vi "生产调试用上位机.vi"() -> ()   [LabVIEW 2016]
uses:
  <vilib>/Utility/miscctls.llb/LVPointTypeDef.ctl
  <vilib>/Utility/config.llb/NI_LVConfig.lvlib
panel:
  in  "隐藏":bool
  out "软件版本":string
  in  "报警查询":bool
  in  "日志查询":bool
  in  "主页按钮":bool
  in  "数据查询":bool
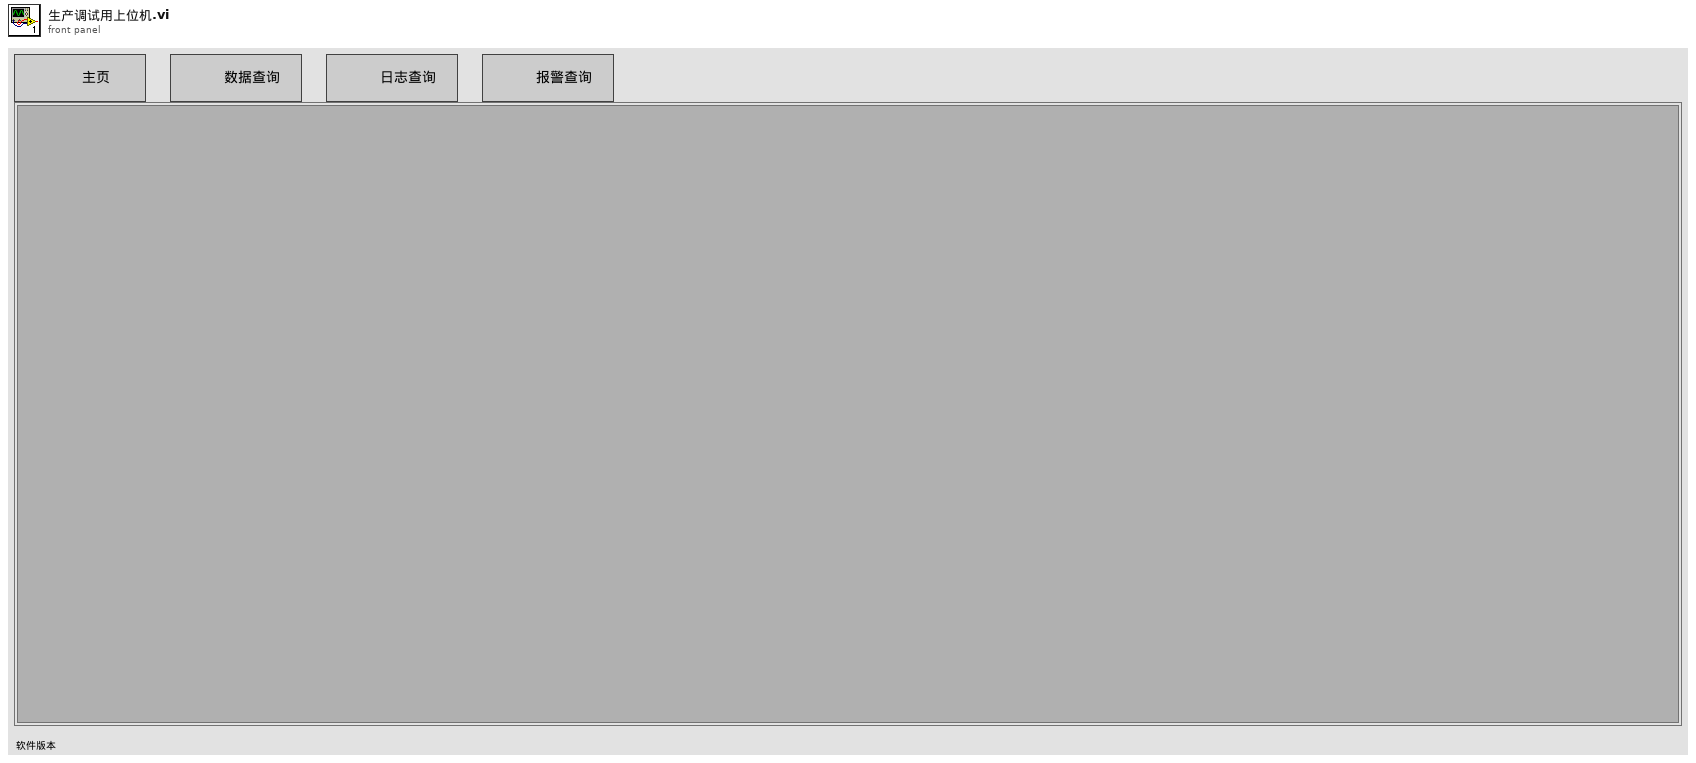
[diagram p1: front panel]
types:
  T1 = typedef "LVPointTypeDef.ctl" = cluster{"Horizontal":i16, "Vertical":i16}
  T2 = typedef "NI_LVConfig.lvlib/Config Data RefNum.ctl" = refnum<k1>
  T3 = enum32{"Bad", "Idle", "Run top level", "Running"}
  T4 = typedef "imagedata.ctl" = cluster{"image type":i32, "image depth":i32, "image":u8[], "mask":u8[], "colors":u32[], "Rectangle":cluster{"left":i16, "top":i16, "right":i16, "bottom":i16}}
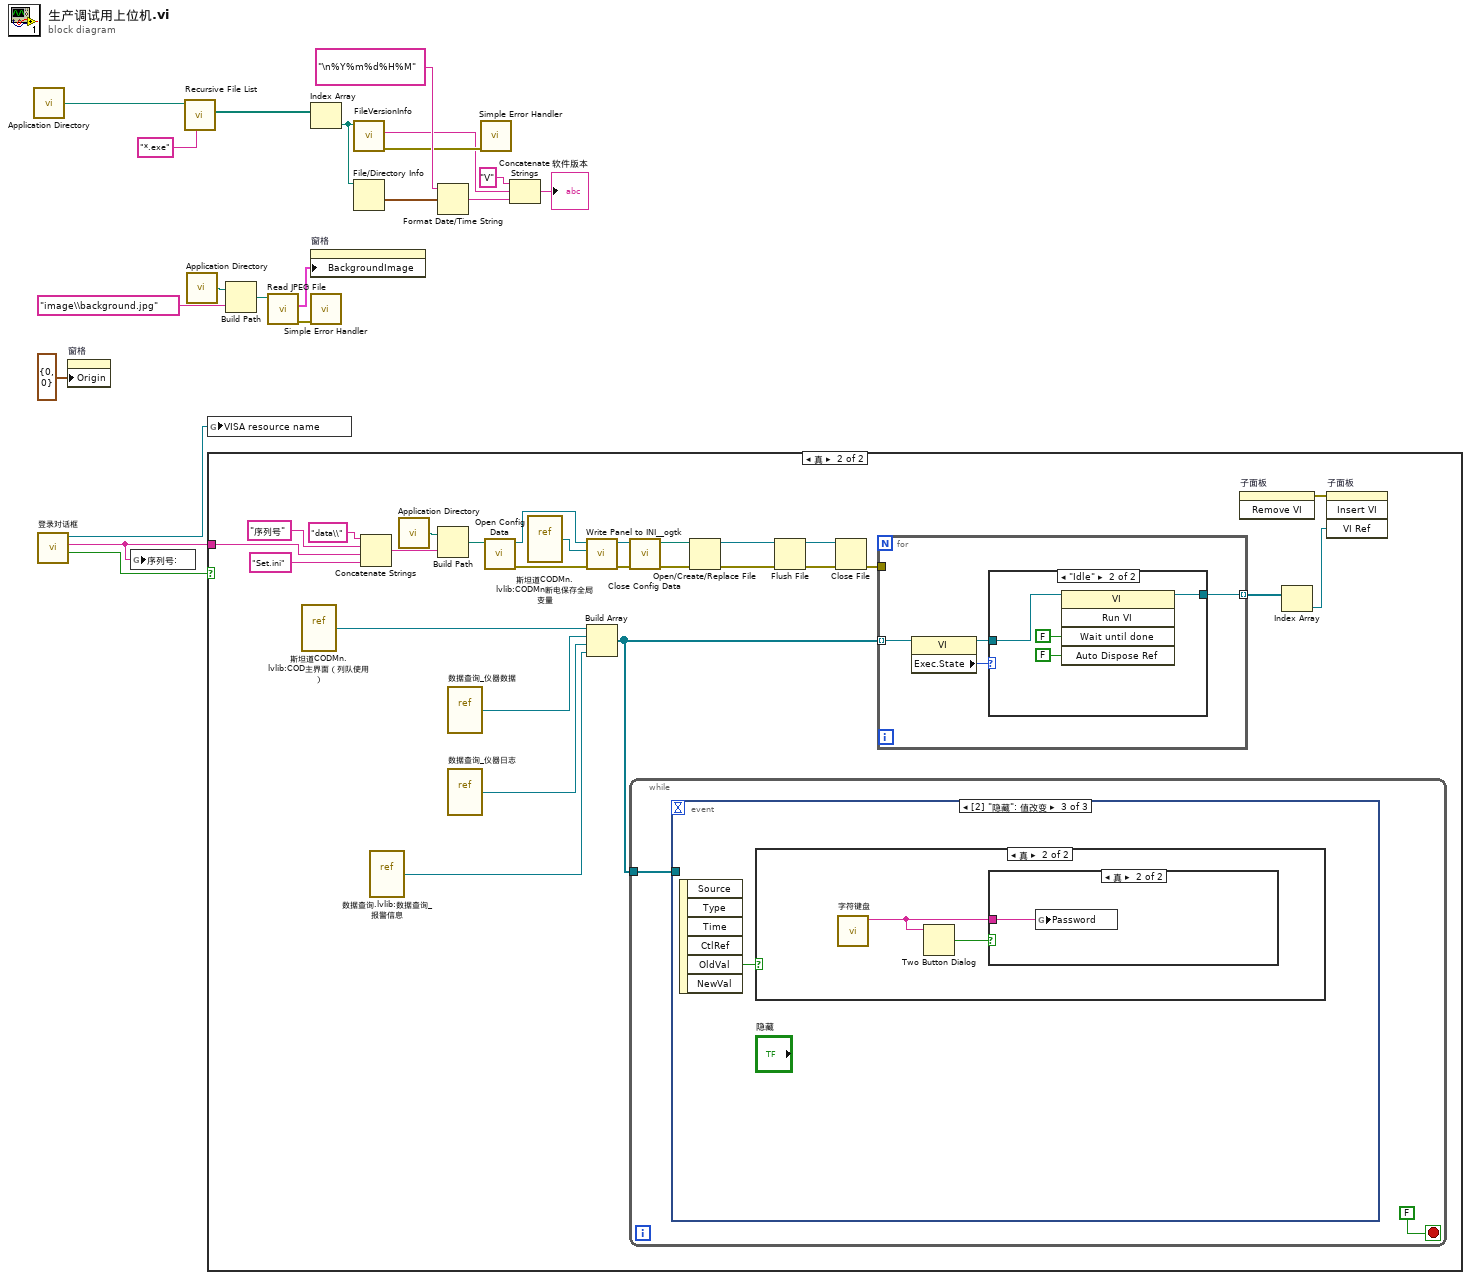
[diagram p0: block diagram]
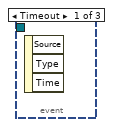
[diagram p4: hidden frame]
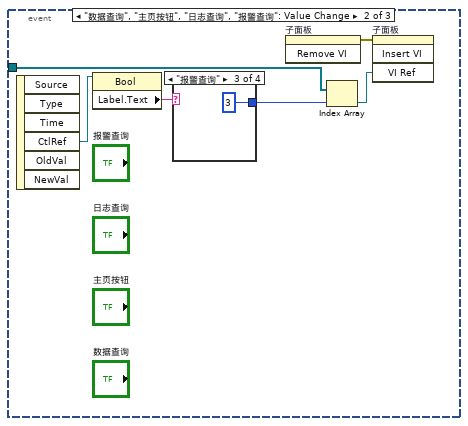
[diagram p5: hidden frame]
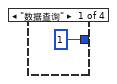
[diagram p6: hidden frame]
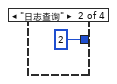
[diagram p7: hidden frame]
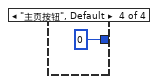
[diagram p8: hidden frame]
diagram:
  n1 = call <vilib>:"Application Directory.vi"() -> ("Application Directory"=w10:path)
  n2 = call "登录对话框.vi"() -> ("输出"=w15:bool, "序列号"=w12:string, "串口号"=w14:refnum<visa-resource-name>)  [unwired: 7 in]
  n3 = property on="窗格" class="Pane"("Origin"=T1 {"Horizontal"=0, "Vertical"=0} ("原点")) -> ()  [unwired: 2 in, 2 out]
  n4 = global write "COD内部交互全局.vi" "序列号:"(w12) -> ()
  n5 = call <vilib>:"Recursive File List.vi"("pattern"="*.exe", "Folder Path"=w10) -> ("All Files in Dir"=w2:path[])  [unwired: 5 in, 4 out]
  n6 = call <vilib>:"Application Directory.vi"() -> ("Application Directory"=w20:path)
  n7 = global write "CODMn断电保存全局变量.vi" "VISA resource name"(w14) -> ()
  n8 = case shown="真" w15 {
    tunnel: w12 -> [_ w38]
    frame False {
    }
    frame True {
      n9 = vi-ref "斯坦道CODMn.lvlib:COD主界面（列队使用）.vi"() -> (w47:refnum<vi>)
      n10 = Concatenate Strings("data\\" ("字符串"), "序列号" ("字符串"), w38, "Set.ini" ("名称或相对路径")) -> (w24:string)
      n11 = vi-ref "数据查询.lvlib:数据查询_报警信息.vi"() -> (w22:refnum<vi>)
      n12 = call <vilib>:"Application Directory.vi"() -> ("Application Directory"=w25:path)
      n13 = Build Path(base path=w25, name or relative path=w24) -> (appended path=w26:path)
      n14 = vi-ref "数据查询_仪器数据.vi"() -> (w46:refnum<vi>)
      n15 = vi-ref "数据查询_仪器日志.vi"() -> (w21:refnum<vi>)
      n16 = call <vilib>:"Open Config Data.vi"("configuration file path"=w26) -> ("error out"=w30:errorcluster, "refnum"=w27:T2)  [unwired: 8 in, 1 out]
      n17 = vi-ref "斯坦道CODMn.lvlib:CODMn断电保存全局变量.vi"() -> (w28:refnum<vi>)
      n18 = call <userlib>:"Write Panel to INI__ogtk.vi"("error in (no error)"=w30, "VI ref"=w28, "refnum"=w27) -> ("error out"=w31:errorcluster, "refnum out"=w29:T2)  [unwired: 7 in]
      n19 = Build Array(w47, w46, w21, w22) -> (w42:refnum<vi>[])
      n20 = call <vilib>:"Close Config Data.vi"("error in (no error)"=w31, "refnum"=w29) -> ("error out"=w36:errorcluster, "file path"=w37:path)  [unwired: 8 in]
      n21 = while {
        tunnel: w42 -> [w57]
        stop <- FALSE stop-if-true
        n22 = event shown="[2] \"隐藏\": 值改变" {
          selector: _ -> [_ _ _]
          dyn-events: _ -> [_ _ _]
          timeout: _ -> [_ _ _]
          tunnel: w57 -> [_ w62 _]
          event Timeout {
            n23 = event-data() -> ()  [unwired: 1 in, 3 out]
          }
          event "数据查询", "主页按钮", "日志查询", "报警查询": Value Change {
            n24 = event-data() -> ("CtlRef"=w61:refnum<vi>)  [unwired: 1 in, 5 out]
            n25 = property class="Bool"(reference=w61) -> ("Label.Text"=w60:string)  [unwired: 1 in, 2 out]
            n26 = case shown="\"报警查询\"" w60 {
              tunnel: [1 ("索引") 2 ("索引") 3 ("索引") 0 ("索引")] -> w59
              frame "数据查询" {
              }
              frame "日志查询" {
              }
              frame "报警查询" {
              }
              frame "主页按钮", Default {
              }
            }
            n27 = invoke on="子面板" class="SubPnl" method="Remove VI"() -> (error out=w63:errorcluster)  [unwired: 3 in, 2 out]
            n28 = Index Array(array=w62, index=w59) -> (element=w64:refnum<vi>)
            n29 = invoke on="子面板" class="SubPnl" method="Insert VI"(error in=w63, "VI Ref"=w64) -> ()  [unwired: 2 in, 4 out]
          }
          event "隐藏": Value Change {
            n30 = event-data() -> ("OldVal"=w69:bool)  [unwired: 1 in, 5 out]
            n31 = case shown="真" w69 {
              frame False {
              }
              frame True {
                n32 = call "字符键盘.vi"() -> ("x+y"=w70:string)  [unwired: 11 in]
                n33 = Two Button Dialog(message=w70) -> (T button?=w71:bool)  [unwired: 2 in]
                n34 = case shown="真" w71 {
                  tunnel: w70 -> [_ w72]
                  frame False {
                  }
                  frame True {
                    n35 = global write "外部调用接口全局变量.vi" "Password"(w72) -> ()
                  }
                }
              }
            }
          }
        }
      }
      n36 = Open/Create/Replace File(file path (use dialog)=w37, error in=w36) -> (refnum out=w33:refnum<file>, error out=w32:errorcluster)  [unwired: 4 in, 1 out]
      n37 = Flush File(refnum=w33, error in=w32) -> (refnum out=w34:refnum<file>, error out=w35:errorcluster)
      n38 = Close File(refnum=w34, error in=w35) -> (error out=w23:errorcluster)  [unwired: 1 out]
      n39 = for {
        tunnel: [w49] -> w44 mode=indexing
        tunnel: w42 -> [w48] mode=indexing
        tunnel: w23 -> [_]
        n40 = property class="VI"(reference=w48) -> (reference out=w50:refnum<vi>, "Exec.State"=w51:T3)  [unwired: 1 in, 1 out]
        n41 = case shown="\"Idle\"" w51 {
          tunnel: w50 -> [w52 w54]
          tunnel: [w52 w53] -> w49
          frame "Bad", Default {
          }
          frame "Idle" {
            n42 = invoke class="VI" method="Run VI"(reference=w54, "Wait until done"=FALSE ("结束前等待"), "Auto Dispose Ref"=FALSE ("自动销毁引用")) -> (reference out=w53:refnum<vi>)  [unwired: 2 in, 4 out]
          }
        }
      }
      n43 = invoke on="子面板" class="SubPnl" method="Remove VI"() -> (error out=w45:errorcluster)  [unwired: 3 in, 2 out]
      n44 = Index Array(array=w44) -> (element=w43:refnum<vi>)  [unwired: 1 in]
      n45 = invoke on="子面板" class="SubPnl" method="Insert VI"(error in=w45, "VI Ref"=w43) -> ()  [unwired: 2 in, 4 out]
    }
  }
  n46 = Build Path(base path=w20, name or relative path="image\\background.jpg" ("名称或相对路径")) -> (appended path=w18:path)
  n47 = call <vilib>:"Read JPEG File.vi"("path to JPEG file"=w18) -> ("error out"=w16:errorcluster, "image data"=w17:T4)  [unwired: 8 in, 1 out]
  n48 = Index Array(array=w2) -> (element=w9:path)  [unwired: 1 in]
  n49 = property on="窗格" class="Pane"("BackgroundImage"=w17) -> ()  [unwired: 2 in, 2 out]
  n50 = call <vilib>:"Simple Error Handler.vi"("error in (no error)"=w16) -> ()  [unwired: 4 in, 5 out]
  n51 = call <vilib>:"FileVersionInfo.vi"("Application Path in"=w9) -> ("error out"=w4:errorcluster, "File Version Info"=w3:string)  [unwired: 7 in, 2 out]
  n52 = File/Directory Info(path=w9) -> (last mod=w8:timestamp)  [unwired: 1 in, 6 out]
  n53 = Format Date/Time String(time format string (%c)="\n%Y%m%d%H%M" ("时间格式字符串(%c)"), seconds (now)=w8) -> (date/time string=w5:string)  [unwired: 1 in]
  n54 = call <vilib>:"Simple Error Handler.vi"("error in (no error)"=w4) -> ()  [unwired: 4 in, 5 out]
  n55 = Concatenate Strings("V" ("字符串"), w3, w5) -> (→"软件版本":string)
